vi "Temperhum.LogPath.vi"(0 "Computer Name":string) -> (9 "Paths":string)   [LabVIEW 2019, in "Instrument.Temperhum.lvclass"]
uses:
  Instrument.Temperhum.lvclass
  <userlib>/LevyLab/LV-Data/LV-Data.PG/LV-Data.PGSQL.lvclass
panel:
  out "error out":errorcluster
  in  "error in (no error)":errorcluster
  out "LV-Data.PGSQL out":refnum<class "LV-Data.PGSQL.lvclass">
  in  "LV-Data.PGSQL":refnum<class "LV-Data.PGSQL.lvclass">
  out "Column Paths":string[](array[string])
  out "Column Names":string[](array[string])
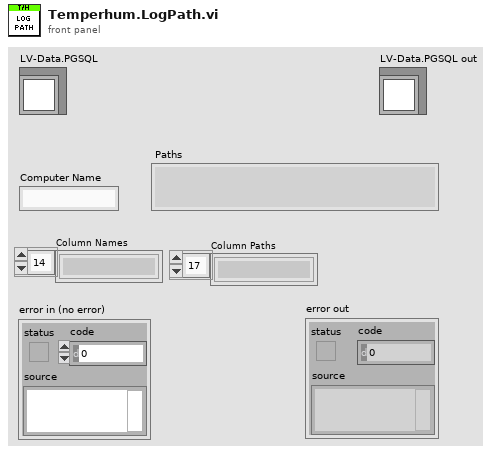
[diagram p1: front panel]
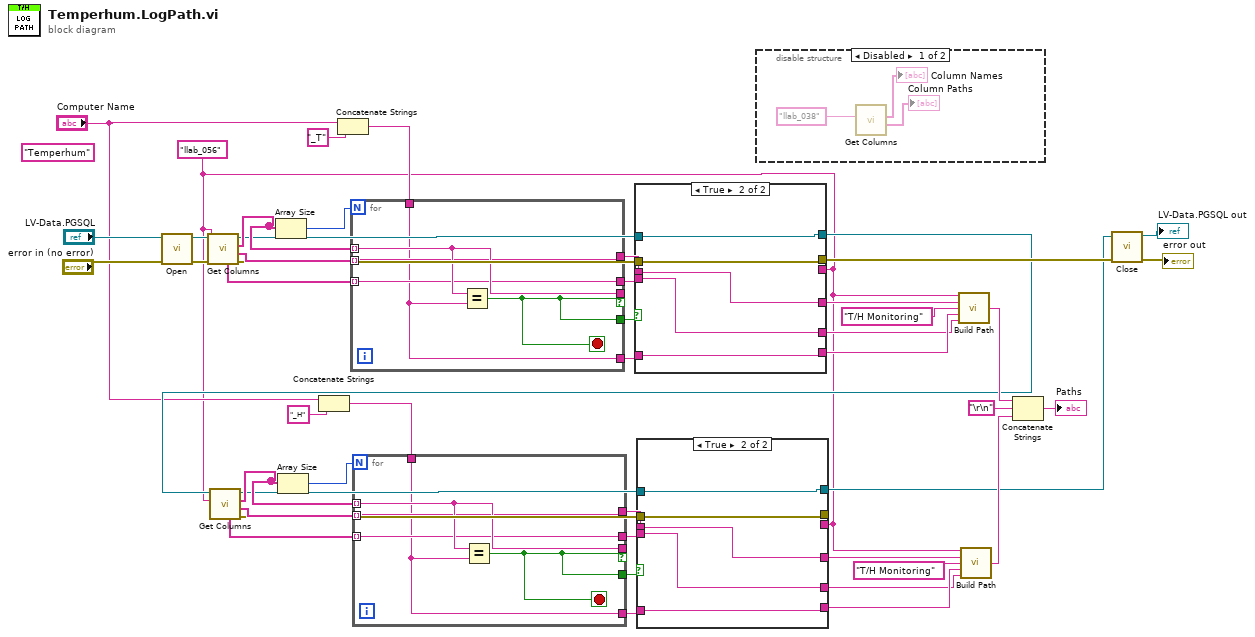
[diagram p0: block diagram]
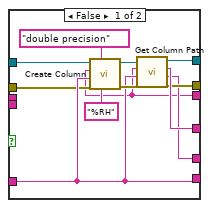
[diagram p3: hidden frame]
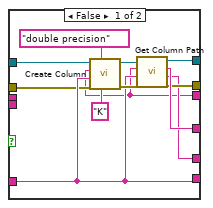
[diagram p4: hidden frame]
diagram:
  (unwired) "Temperhum"
  w1 = "llab_056" ("Table Path")
  n1 = call-dynamic "Open.vi"("error in (no error)"="error in (no error)", "Data.PG in"="LV-Data.PGSQL") -> ("error out"=w35:errorcluster, "Data.PG out"=w12:refnum<class "LV-Data.PGSQL.lvclass">)  [unwired: 8 in]
  n2 = call <userlib>:"Get Columns.vi"("error in (no error)"=w35, "Table Path"=w1, "Data.PG"=w12) -> ("error out"=w31:errorcluster, "Column Paths"=w46:string[], "Column Names"=w36:string[], "Data.PG out"=w34:refnum<class "LV-Data.PGSQL.lvclass">, "Column Units"=w45:string[])  [unwired: 4 in]
  n3 = Array Size(array=w36) -> (size(s)=w47:i32)
  n4 = Concatenate Strings("Computer Name", "_H" ("string")) -> (w9:string)
  n5 = Concatenate Strings("Computer Name", "_T" ("string")) -> (w11:string)
  n6 = for {
    N: w47 -> [_]
    tunnel: w36 -> [w52] mode=indexing
    tunnel: [w52] -> _ if=w51
    tunnel: [w51] -> w43
    tunnel: w46 -> [w50] mode=indexing
    tunnel: [w50] -> w40
    tunnel: [w49] -> w38
    tunnel: w45 -> [w49] mode=indexing
    tunnel: [w48] -> w42
    tunnel: w11 -> [w48]
    stop <- w51 stop-if-true
    n7 = Equal?(x=w52, y=w48) -> (x = y?=w51:bool)
  }
  n8 = case shown="True" w43 {
    tunnel: w42 -> [w61 w69]
    tunnel: [w61 w69] -> w41
    tunnel: w40 -> [_ w68]
    tunnel: [w62 w68] -> w39
    tunnel: [w54 w67] -> w37
    tunnel: w38 -> [_ w67]
    tunnel: w34 -> [w59 w66]
    tunnel: [w57 w66] -> w4
    tunnel: w31 -> [w56 w65]
    tunnel: [w55 w65] -> w27
    tunnel: w1 -> [w53 _]
    frame False {
      n9 = call <userlib>:"Create Column.vi"("new column units"="K", "new column data type"="double precision", "error in (no error)"=w56, "new column name"=w61, "selected table path"=w53, "Data.PGSQL in"=w59) -> ("error out"=w63:errorcluster, "Data.PGSQL out"=w58:refnum<class "LV-Data.PGSQL.lvclass">)  [unwired: 4 in]
      n10 = call <userlib>:"Get Column Path.vi"("error in (no error)"=w63, "Column Name"=w61, "Table path"=w53, "Data.PG in"=w58) -> ("error out"=w55:errorcluster, "Column Unit"=w54:string, "Column Path"=w62:string, "Data.PG out"=w57:refnum<class "LV-Data.PGSQL.lvclass">)  [unwired: 4 in]
    }
    frame True {
    }
  }
  n11 = call <userlib>:"Get Columns.vi"("Table Path"=w1, "Data.PG"=w4) -> ("error out"=w13:errorcluster, "Column Paths"=w25:string[], "Column Names"=w15:string[], "Data.PG out"=w14:refnum<class "LV-Data.PGSQL.lvclass">, "Column Units"=w24:string[])  [unwired: 5 in]
  n12 = Array Size(array=w15) -> (size(s)=w26:i32)
  n13 = for {
    N: w26 -> [_]
    tunnel: w15 -> [w74] mode=indexing
    tunnel: [w74] -> _ if=w73
    tunnel: [w73] -> w22
    tunnel: w25 -> [w72] mode=indexing
    tunnel: [w72] -> w19
    tunnel: [w71] -> w17
    tunnel: w24 -> [w71] mode=indexing
    tunnel: [w70] -> w21
    tunnel: w9 -> [w70]
    stop <- w73 stop-if-true
    n14 = Equal?(x=w74, y=w70) -> (x = y?=w73:bool)
  }
  n15 = case shown="True" w22 {
    tunnel: w21 -> [w83 w91]
    tunnel: [w83 w91] -> w20
    tunnel: w19 -> [_ w90]
    tunnel: [w84 w90] -> w18
    tunnel: [w76 w89] -> w16
    tunnel: w17 -> [_ w89]
    tunnel: w14 -> [w81 w88]
    tunnel: [w79 w88] -> w3
    tunnel: w13 -> [w78 w87]
    tunnel: [w77 w87] -> _
    tunnel: w1 -> [w75 _]
    frame False {
      n16 = call <userlib>:"Create Column.vi"("new column units"="%RH", "new column data type"="double precision", "error in (no error)"=w78, "new column name"=w83, "selected table path"=w75, "Data.PGSQL in"=w81) -> ("error out"=w85:errorcluster, "Data.PGSQL out"=w80:refnum<class "LV-Data.PGSQL.lvclass">)  [unwired: 4 in]
      n17 = call <userlib>:"Get Column Path.vi"("error in (no error)"=w85, "Column Name"=w83, "Table path"=w75, "Data.PG in"=w80) -> ("error out"=w77:errorcluster, "Column Unit"=w76:string, "Column Path"=w84:string, "Data.PG out"=w79:refnum<class "LV-Data.PGSQL.lvclass">)  [unwired: 4 in]
    }
    frame True {
    }
  }
  n18 = disable-structure shown="Disabled" {
    frame Disabled {
      n19 = call <userlib>:"Get Columns.vi"("Table Path"="llab_038") -> ("Column Paths"=→"Column Paths":string[], "Column Names"=→"Column Names":string[])  [unwired: 6 in, 3 out]
    }
    frame Enabled {
    }
  }
  n20 = call <userlib>:"Build Path.vi"("Table path"=w1, "Column path"=w39, "Table name"="T/H Monitoring", "Column name"=w41, "Column units"=w37) -> ("PG path"=w8:string)  [unwired: 10 in]
  n21 = call <userlib>:"Build Path.vi"("Table path"=w1, "Column path"=w18, "Table name"="T/H Monitoring", "Column name"=w20, "Column units"=w16) -> ("PG path"=w5:string)  [unwired: 10 in]
  n22 = Concatenate Strings(w8, "\r\n", w5) -> (→"Paths":string)
  n23 = call-dynamic "Close.vi"("error in (no error)"=w27, "Data.PG in"=w3) -> ("error out"=→"error out":errorcluster, "Data.PG out"=→"LV-Data.PGSQL out":refnum<class "LV-Data.PGSQL.lvclass">)  [unwired: 8 in]
